vi "Write Delay Line Enqueuer.vi"(10 "Actor Framework:Message Enqueuer":refnum<class "Message Enqueuer.lvclass">, 11 "Abstract Controller in":refnum<class "Abstract Controller.lvclass">) -> (3 "Abstract Controller out":refnum<class "Abstract Controller.lvclass">)   [LabVIEW 2016, in "Controllers.lvlib" / "Abstract Controller.lvclass"]
uses:
  Abstract Controller.lvclass
  <vilib>/ActorFramework/Message Enqueuer/Message Enqueuer.lvclass
  Abstract Controller.lvclass/Abstract Controller.ctl
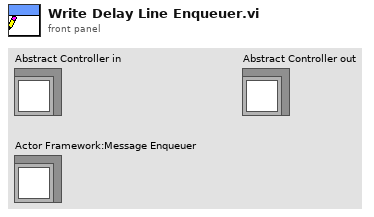
[diagram p1: front panel]
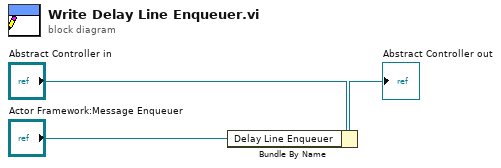
[diagram p0: block diagram]
diagram:
  n1 = Bundle By Name(cluster="Abstract Controller in", "Delay Line Enqueuer"="Actor Framework:Message Enqueuer") -> (→"Abstract Controller out":refnum<class "Abstract Controller.lvclass">)
